vi "20151030 Acc+gyro+kalman filter module.vi"(8 "error in (no error)":errorcluster, 9 "Looptime":u32, 10 "Gyro  Data":T1, 11 "Acceleration Data":T1) -> (0 "error out":errorcluster, 1 "After Kalman filter":T2(graph), 2 "roll":dbl, 3 "pitch":dbl)   [LabVIEW 2013]
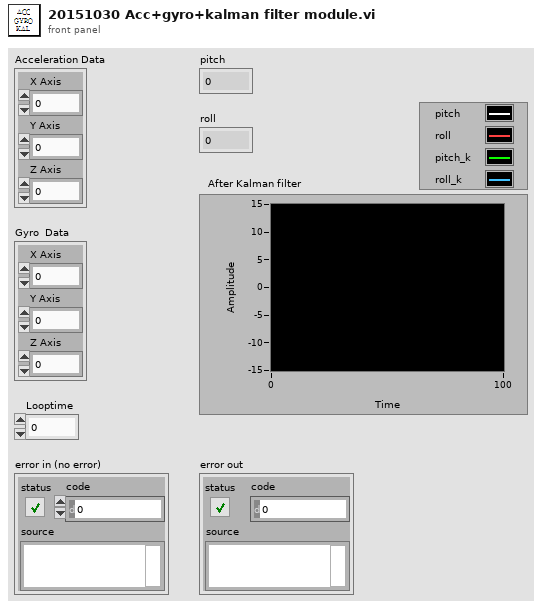
[diagram p1: front panel]
types:
  T1 = cluster{"X Axis":i16, "Y Axis":i16, "Z Axis":i16}
  T2 = cluster{"pitch":dbl, "roll":dbl, "x_angle":dbl, "x_angle":dbl}
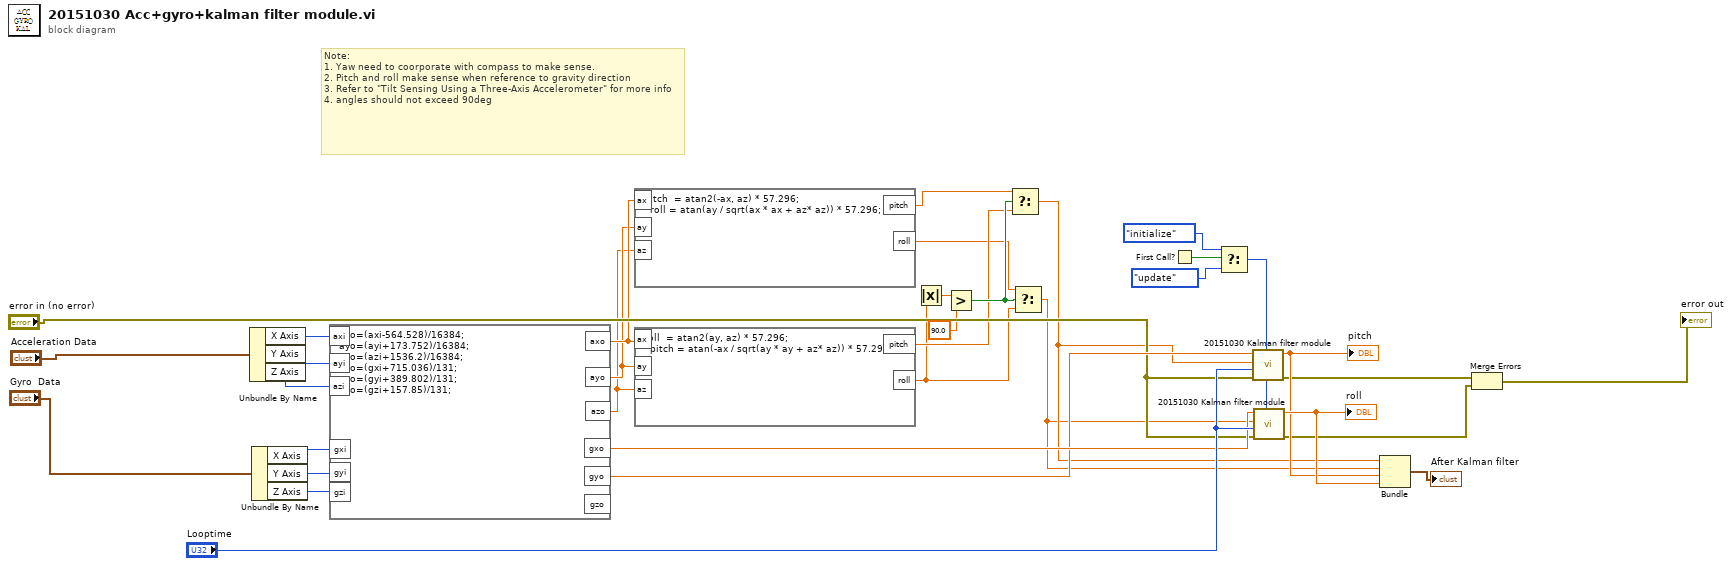
[diagram p0: block diagram]
diagram:
  # "Note: \n1. Yaw need to coorporate with compass to make sense.\n2. Pitch and roll make sense when reference to gravity direction\n3. Refer to \"Tilt Sensing Using a Three-Axis Accelerometer\" for more info\n4. angles should not exceed 90deg"
  # "To pitch and roll"
  # "Calibration\n1. For 2g 250deg/sec"
  n1 = Unbundle By Name("Acceleration Data") -> ("X Axis"=w15:i16, "Y Axis"=w16:i16, "Z Axis"=w17:i16)
  n2 = Unbundle By Name("Gyro  Data") -> ("X Axis"=w18:i16, "Y Axis"=w19:i16, "Z Axis"=w20:i16)
  n3 = formula code="axo=(axi-564.528)/16384;\nayo=(ayi+173.752)/16384;\nazo=(azi+1536.2)/16384;\ngxo=(gxi+715.036)/131;\ngyo=(gyi+389.802)/131;\ngzo=(gzi+157.85)/131;"("axi"=w15, "ayi"=w16, "azi"=w17, "gxi"=w18, "gyi"=w19, "gzi"=w20) -> ("axo"=w12:dbl, "ayo"=w11:dbl, "azo"=w10:dbl, "gxo"=w26:dbl, "gyo"=w25:dbl)  [unwired: 1 out]
  n4 = formula code="pitch  = atan2(-ax, az) * 57.296;\n  roll = atan(ay / sqrt(ax * ax + az* az)) * 57.296;"("ax"=w12, "ay"=w11, "az"=w10) -> ("pitch"=w6:dbl, "roll"=w3:dbl)
  n5 = formula code="roll  = atan2(ay, az) * 57.296;\n  pitch = atan(-ax / sqrt(ay * ay + az* az)) * 57.296;"("ax"=w12, "ay"=w11, "az"=w10) -> ("pitch"=w4:dbl, "roll"=w2:dbl)
  n6 = Absolute Value(x=w2) -> (abs(x)=w9:dbl)
  n7 = Greater?(x=w9, y=90.0) -> (0:w7:bool)
  n8 = Select(t=w6, s=w7, f=w4) -> (s? t:f=w5:dbl)
  n9 = Select(t=w3, s=w7, f=w2) -> (s? t:f=w1:dbl)
  n10 = First Call?() -> (First Call?: T/F=w28:bool)
  n11 = Select(t=enum16{"initialize", "update"}."initialize" ("Action"), s=w28, f=enum16{"initialize", "update"}."update" ("Action")) -> (s? t:f=w31:enum16{"initialize", "update"})
  n12 = call "20151030 Kalman filter module.vi"("Action"=w31, "error in"="error in (no error)", "Looptime"="Looptime", "newAngle"=w5, "newRate"=w25) -> ("error out"=w22:errorcluster, "x_angle"=w32:dbl)  [unwired: 5 in]
  "pitch" <- w32
  n13 = call "20151030 Kalman filter module.vi"("Action"=w31, "error in"="error in (no error)", "Looptime"="Looptime", "newAngle"=w1, "newRate"=w26) -> ("error out"=w23:errorcluster, "x_angle"=w33:dbl)  [unwired: 5 in]
  "roll" <- w33
  n14 = Bundle("pitch"=w5, "roll"=w1, "x_angle"=w32, "x_angle"=w33) -> (→"After Kalman filter":T2)  [unwired: 1 in]
  n15 = Merge Errors(w22, w23) -> (→"error out":errorcluster)
